vi "5492_TwoValveControl.vi"(10 "Button":bool, 11 "SolenoidDevRef":T1={"DevStatus"={"status"=FALSE, "code"=0, "source"=""}, "Pneumatics Control Module"=0, "Forward Solenoid Channel"=enum."Invalid", "Reverse Solenoid Channel"=enum."Invalid"}) -> (3 "SolenoidDevRef 2":T1={"DevStatus"={"status"=FALSE, "code"=0, "source"=""}, "Pneumatics Control Module"=0, "Forward Solenoid Channel"=enum."Invalid", "Reverse Solenoid Channel"=enum."Invalid"})   [LabVIEW 2017]
uses:
  <vilib>/Rock Robotics/WPI/Solenoid/WPI_SolenoidDevRef.ctl
  <vilib>/Rock Robotics/WPI/Solenoid/WPI_SolenoidChannel.ctl
  <vilib>/Rock Robotics/WPI/Solenoid/WPI_SolenoidValue.ctl
  <vilib>/Rock Robotics/WPI/Solenoid/WPI_SolenoidGetEnum.vi
  <vilib>/Rock Robotics/WPI/Solenoid/WPI_SolenoidSetEnum.vi
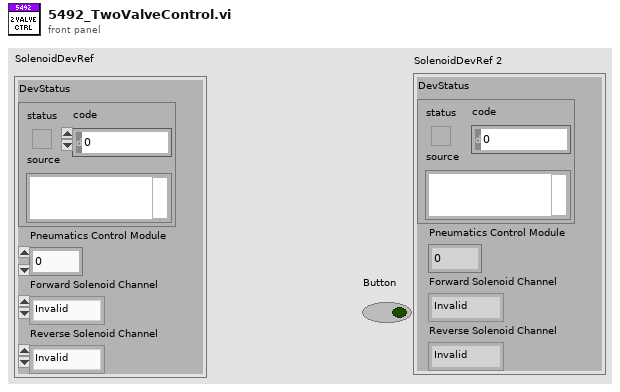
[diagram p1: front panel]
types:
  T1 = typedef "WPI_SolenoidDevRef.ctl" = cluster{"DevStatus":errorcluster, "Pneumatics Control Module":u8, "Forward Solenoid Channel":T2, "Reverse Solenoid Channel":T2}
  T2 = typedef "WPI_SolenoidChannel.ctl" = enum8{"Solenoid 0", "Solenoid 1", "Solenoid 2", "Solenoid 3", "Solenoid 4", "Solenoid 5", "Solenoid 6", "Solenoid 7", "Invalid"}
  T3 = typedef "WPI_SolenoidValue.ctl" = enum16{"Off", "On", "Forward", "Reverse"}
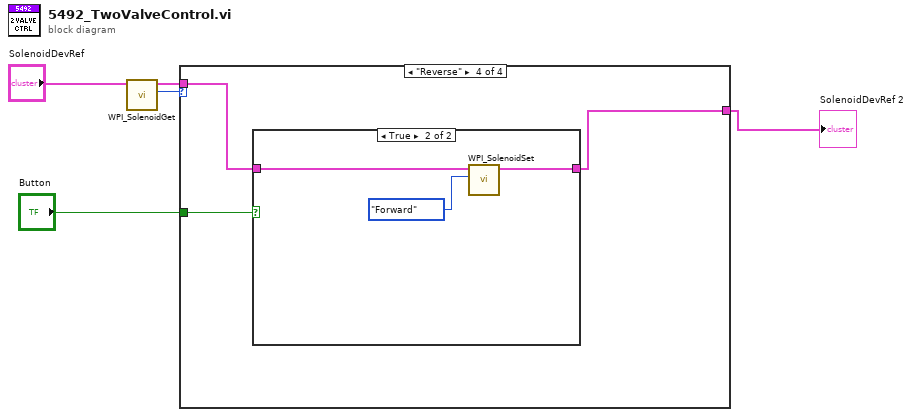
[diagram p0: block diagram]
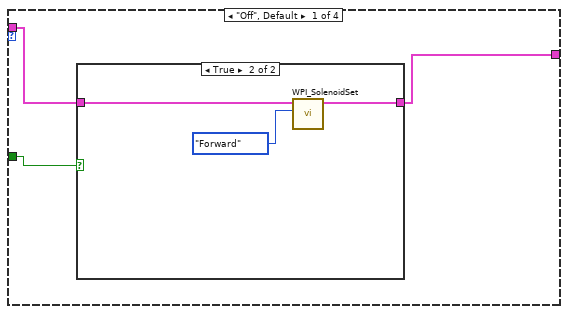
[diagram p2: hidden frame]
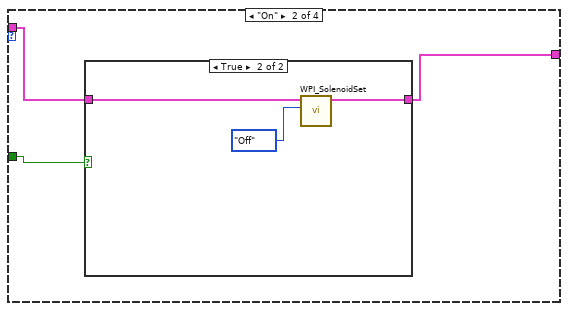
[diagram p4: hidden frame]
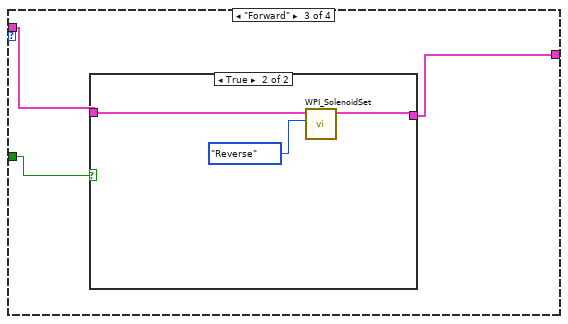
[diagram p6: hidden frame]
diagram:
  n1 = call-poly <vilib>:"WPI_SolenoidGet.vi"("SolenoidDevRef"="SolenoidDevRef") -> ("Value"=w5:T3, "SolenoidDevRef"=w3:T1)  [unwired: 8 in, 1 out]
  n2 = case shown="\"Reverse\"" w5 {
    tunnel: w3 -> [w8 w14 w21 w29]
    tunnel: "Button" -> [w7 w15 w22 w27]
    tunnel: [w6 w13 w20 w28] -> w1
    frame "Off", Default {
      n3 = case shown="True" w7 {
        tunnel: w8 -> [w9 w12]
        tunnel: [w9 w10] -> w6
        frame False {
        }
        frame True {
          n4 = call-poly <vilib>:"WPI_SolenoidSet.vi"("Value"=WPI_SolenoidValue."Forward", "SolenoidDevRef"=w12) -> ("SolenoidDevRef"=w10:T1)  [unwired: 8 in, 1 out]
        }
      }
    }
    frame "On" {
      n5 = case shown="True" w15 {
        tunnel: w14 -> [w16 w19]
        tunnel: [w16 w17] -> w13
        frame False {
        }
        frame True {
          n6 = call-poly <vilib>:"WPI_SolenoidSet.vi"("Value"=WPI_SolenoidValue."Off", "SolenoidDevRef"=w19) -> ("SolenoidDevRef"=w17:T1)  [unwired: 8 in, 1 out]
        }
      }
    }
    frame "Forward" {
      n7 = case shown="True" w22 {
        tunnel: w21 -> [w23 w26]
        tunnel: [w23 w24] -> w20
        frame False {
        }
        frame True {
          n8 = call-poly <vilib>:"WPI_SolenoidSet.vi"("Value"=WPI_SolenoidValue."Reverse", "SolenoidDevRef"=w26) -> ("SolenoidDevRef"=w24:T1)  [unwired: 8 in, 1 out]
        }
      }
    }
    frame "Reverse" {
      n9 = case shown="True" w27 {
        tunnel: w29 -> [w30 w33]
        tunnel: [w30 w31] -> w28
        frame False {
        }
        frame True {
          n10 = call-poly <vilib>:"WPI_SolenoidSet.vi"("Value"=WPI_SolenoidValue."Forward", "SolenoidDevRef"=w33) -> ("SolenoidDevRef"=w31:T1)  [unwired: 8 in, 1 out]
        }
      }
    }
  }
  "SolenoidDevRef 2" <- w1
